vi "IGcontrolLogic.vi"(0 "Ion Gauge Control":T2, 1 "CG Safety Threshold":dbl, 2 "In shot time window":bool, 3 "IG Select":bool, 4 "Vacuum Sensors":T3={"TP On"=FALSE, "IG1 On"=TRUE, "IG2On"=FALSE, "IG Vac Level"=7.206095277894153e-07, "CG1 Vac Level"=7.188197481794052e-05, "CG2 Vac Level"=7.698533430214743e-05, "IG Status"=TRUE} {"CG2 Vac Level" format="%#_2e"; "CG1 Vac Level" format="%#_2e"; "IG Vac Level" format="%#_2e"}) -> (5 "Vacuum Status":T1={"Vacuum Sensors"={"TP On"=FALSE, "IG1 On"=TRUE, "IG2On"=FALSE, "IG Vac Level"=7.206095277894153e-07, "CG1 Vac Level"=7.188197481794052e-05, "CG2 Vac Level"=7.698533430214743e-05, "IG Status"=TRUE}, "In Shot Time Window"=FALSE, "IG reading meaningful"=FALSE} {"Vacuum Sensors"."CG2 Vac Level" format="%#_2e"; "Vacuum Sensors"."CG1 Vac Level" format="%#_2e"; "Vacuum Sensors"."IG Vac Level" format="%#_2e"}, 6 "CG Pressure Safe":bool, 7 "IG should turn on":bool)   [LabVIEW 2016]
uses:
  VacuumMeasurementControlState.ctl
  VacuumStatus.ctl
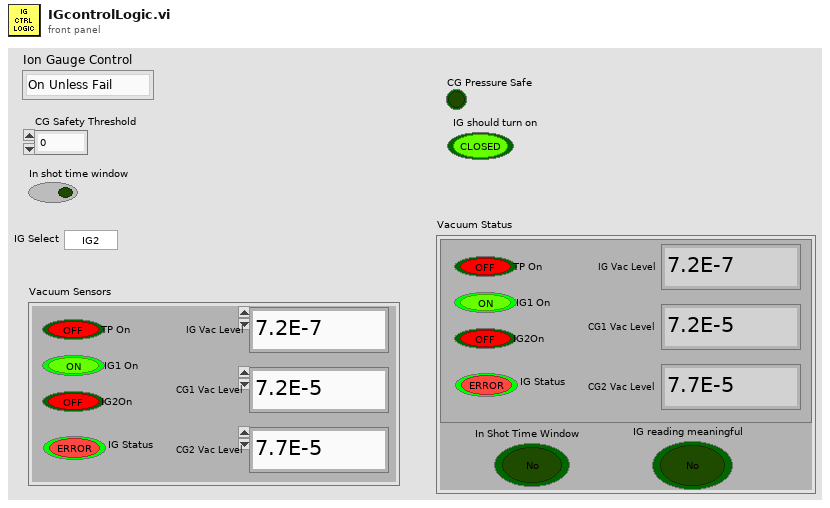
[diagram p1: front panel]
types:
  T1 = typedef "VacuumStatus.ctl" = cluster{"Vacuum Sensors":cluster{"TP On":bool, "IG1 On":bool, "IG2On":bool, "IG Vac Level":dbl, "CG1 Vac Level":dbl, "CG2 Vac Level":dbl, "IG Status":bool}, "In Shot Time Window":bool, "IG reading meaningful":bool}
  T2 = typedef "VacuumMeasurementControlState.ctl" = enum16{"On Unless Fail", "On Unless Shot", "Force Off", "Manual"}
  T3 = cluster{"TP On":bool, "IG1 On":bool, "IG2On":bool, "IG Vac Level":dbl, "CG1 Vac Level":dbl, "CG2 Vac Level":dbl, "IG Status":bool}
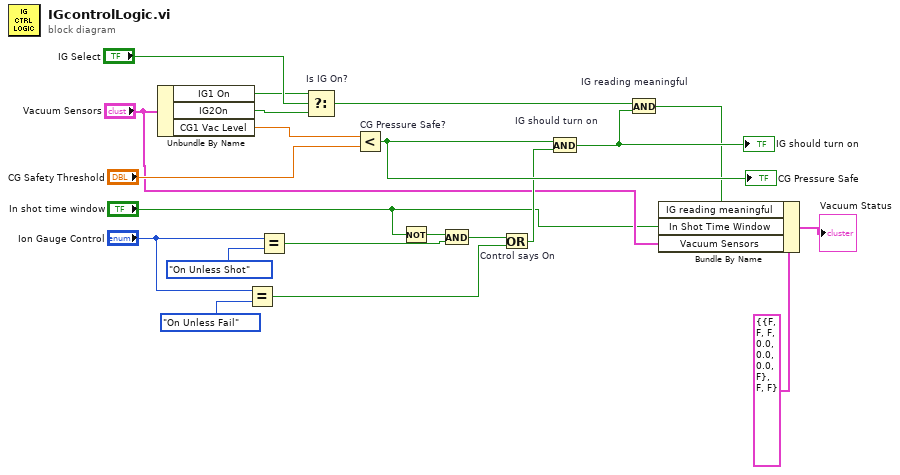
[diagram p0: block diagram]
diagram:
  n1 = Unbundle By Name("Vacuum Sensors") -> ("IG1 On"=w9:bool, "IG2On"=w8:bool, "CG1 Vac Level"=w21:dbl)
  n2 = Equal?(x="Ion Gauge Control", y=VacuumMeasurementControlState."On Unless Fail") -> (x = y?=w13:bool)
  n3 = Equal?(x="Ion Gauge Control", y=VacuumMeasurementControlState."On Unless Shot") -> (x = y?=w16:bool)
  n4 = Select "Is IG On?"(t=w9, s="IG Select", f=w8) -> (s? t:f=w6:bool)
  n5 = Less? "CG Pressure Safe?"(x=w21, y="CG Safety Threshold") -> (x < y?=w12:bool)
  "CG Pressure Safe" <- w12
  n6 = Not(x="In shot time window") -> (.not. x?=w15:bool)
  n7 = And(x=w15, y=w16) -> (x .and. y?=w14:bool)
  n8 = Or "Control says On"(x=w14, y=w13) -> (x .or. y?=w11:bool)
  n9 = And "IG should turn on"(x=w12, y=w11) -> (x .and. y?=w7:bool)
  "IG should turn on" <- w7
  n10 = And "IG reading meaningful"(x=w6, y=w7) -> (x .and. y?=w2:bool)
  n11 = Bundle By Name(cluster=T1 {"Vacuum Sensors"={"TP On"=FALSE, "IG1 On"=FALSE, "IG2On"=FALSE, "IG Vac Level"=0.0, "CG1 Vac Level"=0.0, "CG2 Vac Level"=0.0, "IG Status"=FALSE}, "In Shot Time Window"=FALSE, "IG reading meaningful"=FALSE} ("Vacuum Status"), "IG reading meaningful"=w2, "In Shot Time Window"="In shot time window", "Vacuum Sensors"="Vacuum Sensors") -> (→"Vacuum Status":T1)
